vi "Build EthernetFrame (UDP).vi"(10 "UDP header":T1, 11 "Ethernet Frame In":u8[](array[numeric]) format="%.0x") -> (3 "Ethernet Frame Out":u8[](array[numeric]) format="%.0x")   [LabVIEW 2020, in "EthFrameManagement.lvlib"]
uses:
  EthFrameManagement.lvlib
  controls/UDPFrame_type.ctl
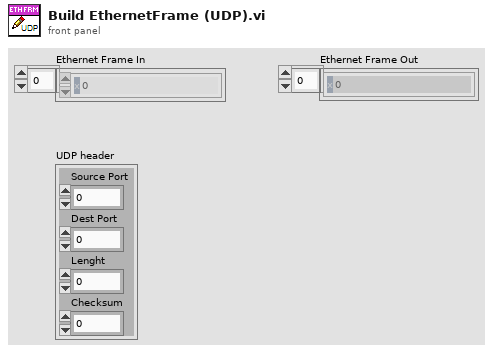
[diagram p1: front panel]
types:
  T1 = typedef "EthFrameManagement.lvlib/UDPFrame_type.ctl" = cluster{"Source Port":u16, "Dest Port":u16, "Lenght":u16, "Checksum":u16}
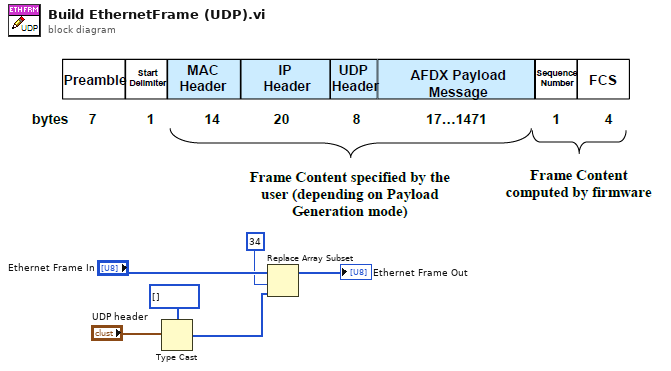
[diagram p0: block diagram]
diagram:
  n1 = Type Cast(type=u8[] [] ("Ethernet Frame In"), x="UDP header") -> (*(type *) &x=w2:u8[])
  n2 = Replace Array Subset(array="Ethernet Frame In", new element=w2, index=34) -> (→"Ethernet Frame Out":u8[])
